vi "DisableAllMarkers.vi"(8 "error in (no error)":errorcluster, 11 "Keysight44xx in":refnum<class "Keysight44xx.lvclass">) -> (0 "error out":errorcluster, 3 "Keysight44xx out":refnum<class "Keysight44xx.lvclass">)   [LabVIEW 2018, in "SpecAnPlugins.lvlib" / "Keysight44xx.lvclass"]
doc: "This VI turns off all the markers."
uses:
  Keysight44xx.lvclass
  C:/Users/ico/Documents/Projects/NistPluggableModules/SpecAn/SpecAnPlugins/SpecAnBaseClass/SpecAnBase.lvclass
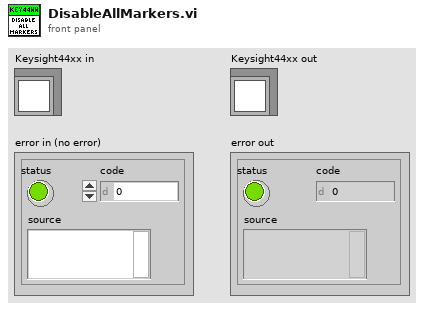
[diagram p1: front panel]
types:
  T1 = typedef "SpecAnPlugins.lvlib/SpecAnBase.lvclass/Acquisition.ctl" = cluster{"Handle":string, "Connected":bool, "Enabled":bool, "SweepModeContinuous":bool, "NumberOfSweeps":i32, "DetectorTypeAuto":bool, "DetectorType":i32, "VerticalScale":i32, "MaximumTime(seconds)":dbl}
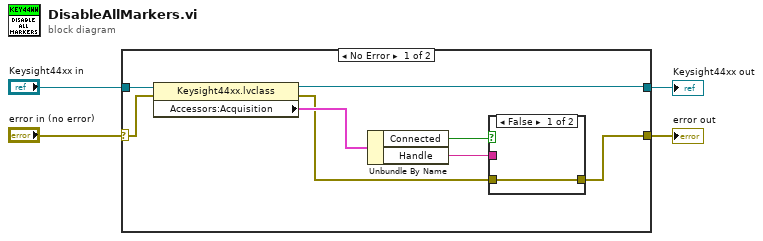
[diagram p0: block diagram]
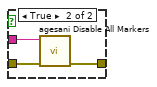
[diagram p2: hidden frame]
diagram:
  n1 = case shown="No Error" "error in (no error)" {
    selector: "error in (no error)" -> [w11 w17]
    tunnel: "Keysight44xx in" -> [w12 w18]
    tunnel: [w10 w18] -> w2
    tunnel: [w6 w17] -> w1
    frame No Error {
      n2 = property class="Keysight44xx.lvclass"(reference=w12, error in=w11) -> (reference out=w10:refnum<class "Keysight44xx.lvclass">, error out=w7:errorcluster, "Accessors:Acquisition"=w9:T1)
      n3 = Unbundle By Name(w9) -> ("Connected"=w5:bool, "Handle"=w8:string)
      n4 = case shown="False" w5 {
        tunnel: w8 -> [_ w16]
        tunnel: w7 -> [w13 w15]
        tunnel: [w13 w14] -> w6
        frame False {
        }
        frame True {
          n5 = call <instrlib>:"agesani Disable All Markers.vi"("error in (no error)"=w15, "instrument handle"=w16) -> ("error out"=w14:errorcluster)  [unwired: 8 in, 1 out]
        }
      }
    }
    frame Error {
    }
  }
  "error out" <- w1
  "Keysight44xx out" <- w2
